vi "Stop Core.vi"(10 "final error code":i32, 11 "Multiharp in":refnum<class "Multiharp.lvclass">) -> (3 "Multiharp out":refnum<class "Multiharp.lvclass">)   [LabVIEW 2023, in "Multiharp.lvlib" / "Multiharp.lvclass"]
doc: "(<B>Filename</B>: Actor Framework.lvlib:Actor.lvclass:Stop Core.vi)\n\nDefines what the actor does before it stops. Use the <B>final error code</B> input to determine whether the actor shut down in response to an error.\n\nBy default, this method passes the Stop message along to all auto-stop nested actors. A descendant class may override this method to define additional behavior, such as shutting down any processes the actor initiated in its override of the Actor Core method."
uses:
  Multiharp.lvclass
  <vilib>/ActorFramework/Actor/Actor.lvclass
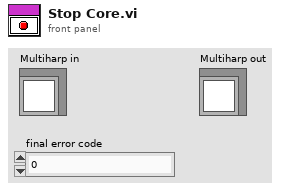
[diagram p1: front panel]
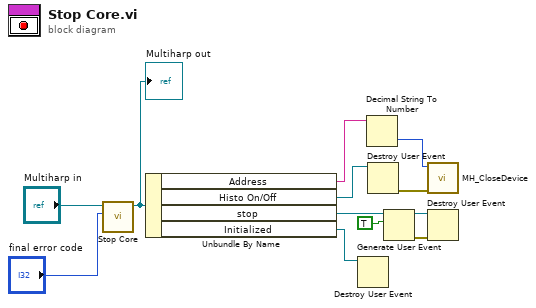
[diagram p0: block diagram]
diagram:
  n1 = call-parent "Stop Core.vi"("final error code"="final error code", "Actor in"="Multiharp in") -> ("Actor out"=w10:refnum<class "Multiharp.lvclass">)  [unwired: 9 in]
  "Multiharp out" <- w10
  n2 = Unbundle By Name(w10) -> ("Address"=w9:string, "Histo On/Off"=w7:refnum<user-event>, "stop"=w4:refnum<user-event>, "Initialized"=w1:refnum<user-event>)
  n3 = Destroy User Event(user event=w1) -> ()  [unwired: 1 in, 1 out]
  n4 = Decimal String To Number(string=w9) -> (number=w8:i32)  [unwired: 2 in, 1 out]
  n5 = Destroy User Event(user event=w7) -> (error out=w6:errorcluster)  [unwired: 1 in]
  n6 = Generate User Event(user event=w4, event data cluster=TRUE ("event data")) -> (user event out=w2:refnum<user-event>, error out=w5:errorcluster)  [unwired: 2 in]
  n7 = call "MH_CloseDevice.vi"("error in (no error)"=w6, "devidx"=w8) -> ()  [unwired: 8 in, 2 out]
  n8 = Destroy User Event(user event=w2, error in=w5) -> ()  [unwired: 1 out]
